vi "IncrementSCMElement.vi"(7 "Decrement? (F)":bool, 11 "ID in":T1) -> (3 "ID out":T1)   [LabVIEW 2016]
uses:
  <vilib>/addons/Software Calibration Management/xSCM/Controls/ID and Element.ctl
  <vilib>/addons/Software Calibration Management/xSCM/SCM-API.lvlib
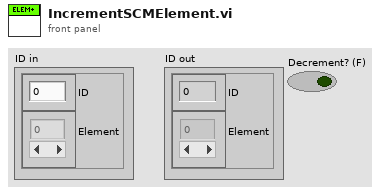
[diagram p1: front panel]
types:
  T1 = typedef "SCM-API.lvlib/ID and Element.ctl" = cluster{"ID":u32, "Element":i32[]}
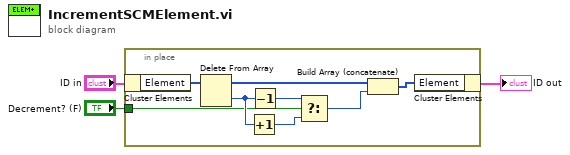
[diagram p0: block diagram]
diagram:
  n1 = in-place {
    in-place-border: "Decrement? (F)" -> [w4]
    n2 = in-place-cluster #1("ID in") -> ("Element"=w11:i32[])
    n3 = Delete From Array(array=w11) -> (deleted portion=w6:i32, array with subset deleted=w10:i32[])  [unwired: 2 in]
    n4 = Increment(x=w6) -> (x+1=w7:i32)
    n5 = Decrement(x=w6) -> (x-1=w8:i32)
    n6 = Select(t=w8, s=w4, f=w7) -> (s? t:f=w5:i32)
    n7 = Build Array (concatenate)(w10, w5) -> (w9:i32[])
    n8 = in-place-cluster #1("Element"=w9) -> (→"ID out":T1)
  }
